vi "read_params.vi"(8 "error in (no error)":errorcluster, 11 "RadiusNeighborsClassifier in":refnum<class "RadiusNeighborsClassifier.lvclass">) -> (0 "error out":errorcluster, 2 "params":T1={"radius"=1.0, "weights"="uniform", "algorithm"="auto", "leaf_size"=30.0, "p"=2.0, "metric"="minkowski", "outlier_label"={"outlier_label_type"="None", "outlier_label_str"="outlier", "outlier_label_int"=-1.0, "outlier_label_list"=[]}, "n_jobs"=1.0}, 3 "RadiusNeighborsClassifier out":refnum<class "RadiusNeighborsClassifier.lvclass">)   [LabVIEW 2020, in "RadiusNeighborsClassifier.lvclass"]
uses:
  RadiusNeighborsClassifier.lvclass
  Controls/radius_neighbors_classifier_params.ctl
  RadiusNeighborsClassifier.lvclass/RadiusNeighborsClassifier.ctl
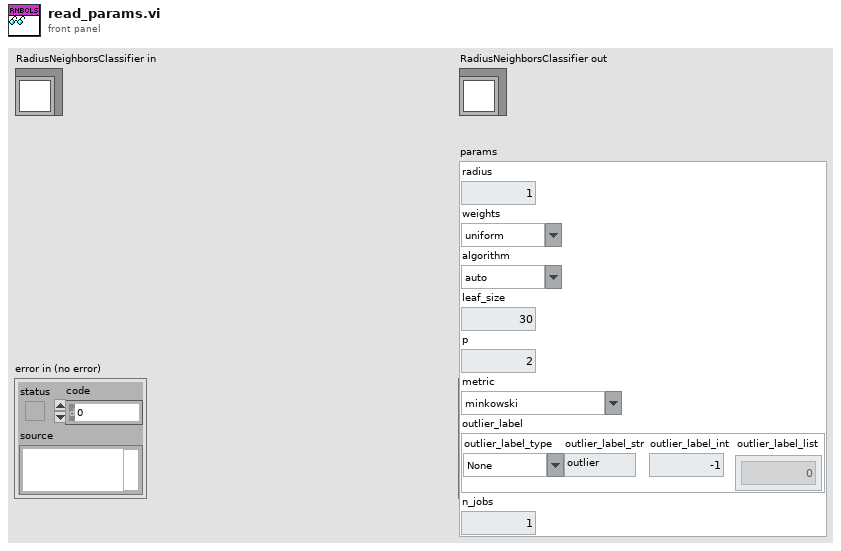
[diagram p1: front panel]
types:
  T1 = typedef "radius_neighbors_classifier_params.ctl" = cluster{"radius":dbl, "weights":string, "algorithm":string, "leaf_size":dbl, "p":dbl, "metric":string, "outlier_label":cluster{"outlier_label_type":string, "outlier_label_str":string, "outlier_label_int":dbl, "outlier_label_list":dbl[]}, "n_jobs":dbl}
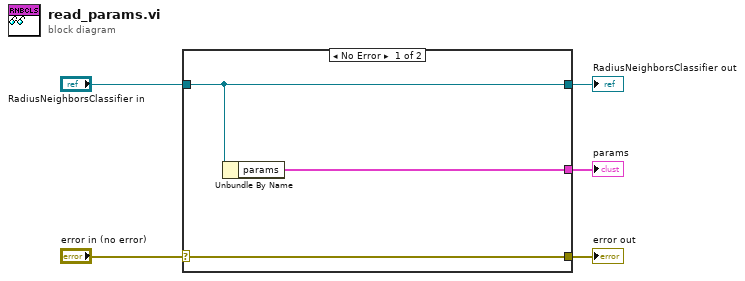
[diagram p0: block diagram]
diagram:
  n1 = case shown="No Error" "error in (no error)" {
    selector: "error in (no error)" -> [w8 w9]
    tunnel: [w8 w9] -> w4
    tunnel: [w7 w10] -> w2
    tunnel: "RadiusNeighborsClassifier in" -> [w7 w10]
    tunnel: [w6 _] -> w1
    frame No Error {
      n2 = Unbundle By Name(w7) -> ("params"=w6:T1)
    }
    frame Error {
    }
  }
  "error out" <- w4
  "RadiusNeighborsClassifier out" <- w2
  "params" <- w1
